vi "Set Start Trigger (Start Immediately).vi"(5 "Retriggerable (F)":bool, 8 "error in (no error)":errorcluster, 11 "Data Logging Specification Ref in":T1) -> (0 "error out":errorcluster, 3 "Data Logging Specification Ref out":T1)   [LabVIEW 2020, in "NI_VS Data Logging API.lvlib"]
doc: "Specifies a trigger condition on which to start logging data. You also can specify whether to log channel data immediately preceding the trigger condition and whether logging is retriggerable, meaning the data logging session watches for subsequent occurrences of the start trigger after the first logging operation finishes. By default, logging stops after one operation.\n\nYou must manually select the polymorphic instance to use."
uses:
  <vilib>/NI VeriStand/Execution/DataLogging/NI_VS Data Logging API.lvlib
  <vilib>/NI VeriStand/Execution/DataLogging/DataLoggingSpecification Ref.ctl
  NationalInstruments.VeriStand.ClientAPI
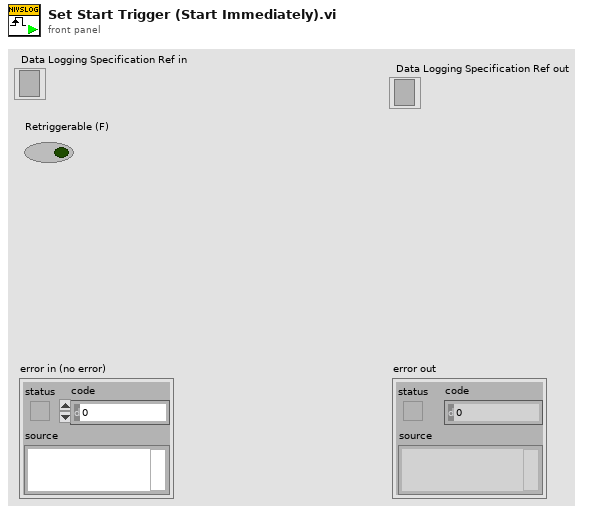
[diagram p1: front panel]
types:
  T1 = typedef "NI_VS Data Logging API.lvlib/DataLoggingSpecification Ref.ctl" = refnum<k24>
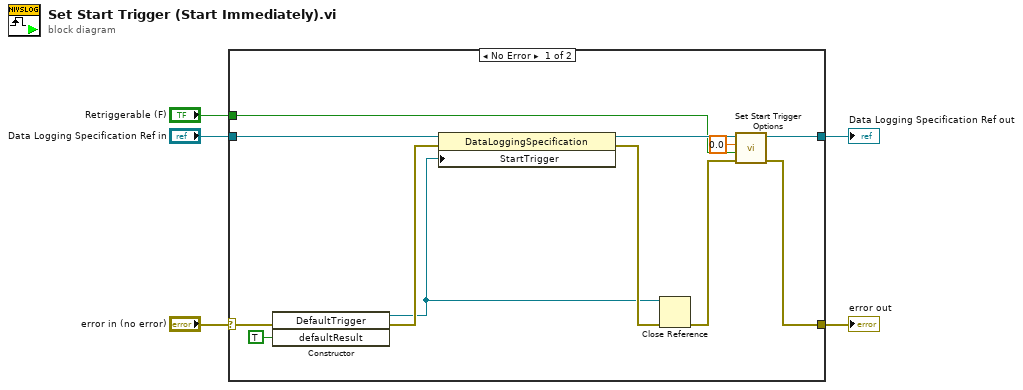
[diagram p0: block diagram]
diagram:
  n1 = case shown="No Error" "error in (no error)" {
    selector: "error in (no error)" -> [w10 w19]
    tunnel: "Data Logging Specification Ref in" -> [w15 w18]
    tunnel: [w12 w18] -> w4
    tunnel: [w11 w19] -> w3
    tunnel: "Retriggerable (F)" -> [w7 _]
    frame No Error {
      n2 = constructor class="DefaultTrigger"(error in=w10, "defaultResult"=TRUE) -> (reference out=w9:refnum<k24>, error out=w17:errorcluster)  [unwired: 2 in, 2 out]
      n3 = property class="DataLoggingSpecification"(reference=w15, error in=w17, "StartTrigger"=w9) -> (reference out=w14:T1, error out=w16:errorcluster)
      n4 = Close Reference(reference=w9, error in (no error)=w16) -> (error out=w13:errorcluster)
      n5 = call <vilib>:"Set Start Trigger Options.vi"("error in (no error)"=w13, "Retriggerable"=w7, "Pre-Trigger Duration"=0.0, "Data Logging Specification Ref in"=w14) -> ("error out"=w11:errorcluster, "Data Logging Specification Ref out"=w12:T1)  [unwired: 6 in]
    }
    frame Error {
    }
  }
  "error out" <- w3
  "Data Logging Specification Ref out" <- w4
